vi "ModeMgr.Load Mode Config.vi"(6 "Options":string[](array[string])=["Display Result Data Details", "Not Reset SN between Tests", "Not Validate Operator", "Not Validate SN", "Disable Results", "Can Access Station Module", "Can Edit EQ List", "Can Clear Warnings", "Can Clear Errors", "Can View Config", "Can Edit Options", "Can Select Sequence", "Can Generate Reports", "Disable Start with SN Entry", "Can Auto Repeat Sequence"], 8 "Use DIalog":bool, 9 "Path":path, 10 "Modes":T1[](array[typedef]) {"Color" items=["Red", "Yellow", "Orange", "Green", "SkyBlue", "Blue", "Purple", "Pink", "Grey"]}, 11 "Default Mode":string="Production") -> (0 "error out":errorcluster, 1 "Names":string[](array[string]), 2 "Modes Out":T1[](array[typedef]) {"Color" items=["Red", "Yellow", "Orange", "Green", "SkyBlue", "Blue", "Purple", "Pink", "Grey"]}, 3 "Default Mode Out":string="Production")   [LabVIEW 2018]
uses:
  ModeMgr.Mode Settings_Config View.ctl
  ModeMgr.Mode Settings.ctl
  ModeMgr.ModeConfig.ctl
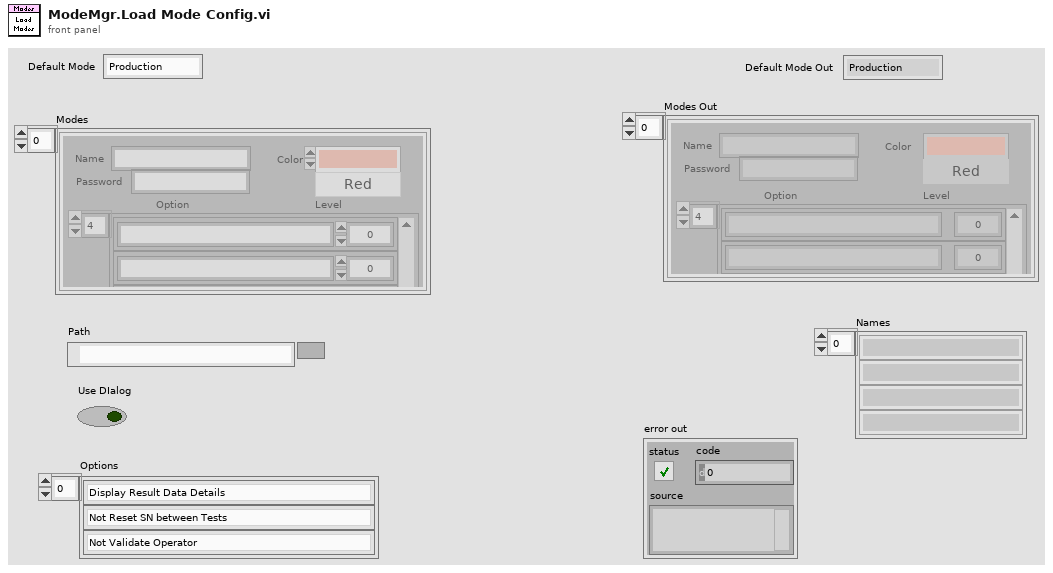
[diagram p1: front panel]
types:
  T1 = typedef "ModeMgr.Mode Settings_Config View.ctl" = cluster{"Name":string, "Color":u16, "Options":T2[], "Password":string}
  T2 = typedef "ModeMgr.Mode Settings.ctl" = cluster{"Option":string, "Level":i32}
  T3 = typedef "ModeMgr.ModeConfig.ctl" = cluster{"Name":string, "Color":string, "Settings":T2[], "Password":string}
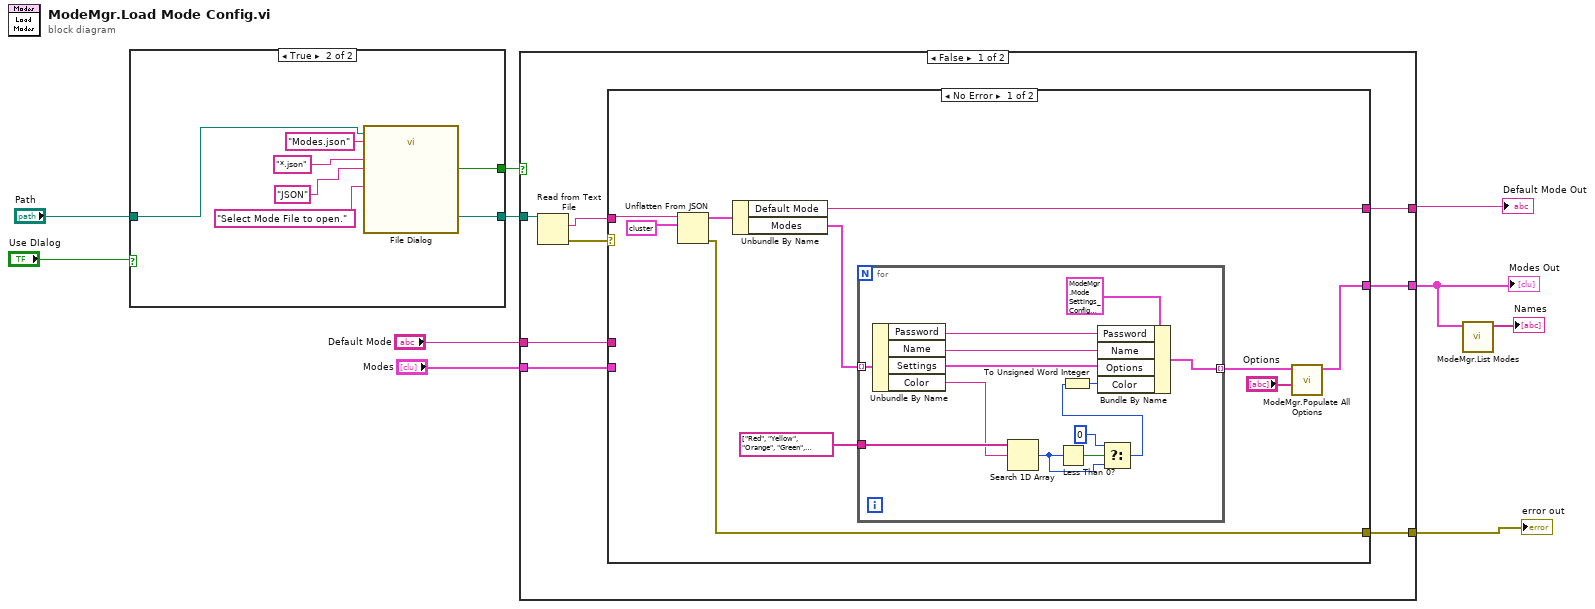
[diagram p0: block diagram]
diagram:
  n1 = case shown="True" "Use DIalog" {
    tunnel: [w11 w14] -> w10
    tunnel: "Path" -> [w11 w13]
    tunnel: [_ w12] -> w8
    frame False {
    }
    frame True {
      n2 = call "File Dialog"("start path"=w13, "prompt"="Select Mode File to open." ("prompt (Choose or enter file path)"), "default name"="Modes.json", "pattern (all files)"="*.json", "pattern label"="JSON" ("pattern (all files)")) -> ("selected path"=w14:path, "cancelled"=w12:bool)  [unwired: 7 in, 2 out]
    }
  }
  n3 = case shown="False" w8 {
    tunnel: w10 -> [w25 _]
    tunnel: [w24 w53] -> w6
    tunnel: [w23 w52] -> w3
    tunnel: "Default Mode" -> [w22 w53]
    tunnel: "Modes" -> [w21 w52]
    tunnel: [w19 _] -> w1
    frame False {
      n4 = Read from Text File(file (use dialog)=w25) -> (text=w26:string, error out=w20:errorcluster)  [unwired: 3 in, 2 out]
      n5 = case shown="No Error" w20 {
        tunnel: w26 -> [w36 _]
        tunnel: [w31 _] -> w19
        tunnel: [w29 w51] -> w24
        tunnel: [w27 w50] -> w23
        tunnel: w22 -> [_ w51]
        tunnel: w21 -> [_ w50]
        frame No Error {
          n6 = Unflatten From JSON(JSON string=w36, type and defaults=cluster{"Default Mode":string, "Modes":T3[]} {"Default Mode"="Production", "Modes"=[{"Name"="Production", "Color"="Green", "Settings"=[{"Option"="PreTest_Validate_SN", "Level"=1}, {"Option"="PostTest_ReportResult", "Level"=1}, {"Option"="OptTo_NotSaveResults", "Level"=0}, {"Option"="OptTo_NotStopOnFail", "Level"=0}, {"Option"="OptTo_SetConfig", "Level"=0}, {"Option"="OptTo_UpdateEquipmentList", "Level"=0}, {"Option"="OptTo_AccessManualStaControl", "Level"=0}], "Password"=""}, {"Name"="Technician", "Color"="Yellow", "Settings"=[{"Option"="PreTest_Validate_SN", "Level"=0}, {"Option"="PostTest_ReportResult", "Level"=0}, {"Option"="OptTo_NotSaveResults", "Level"=1}, {"Option"="OptTo_NotStopOnFail", "Level"=1}, {"Option"="OptTo_SetConfig", "Level"=0}, {"Option"="OptTo_UpdateEquipmentList", "Level"=0}, {"Option"="OptTo_AccessManualStaControl", "Level"=0}], "Password"=""}, {"Name"="Engineering", "Color"="SkyBlue", "Settings"=[{"Option"="PreTest_Validate_SN", "Level"=0}, {"Option"="PostTest_ReportResult", "Level"=0}, {"Option"="OptTo_NotSaveResults", "Level"=1}, {"Option"="OptTo_NotStopOnFail", "Level"=1}, {"Option"="OptTo_SetConfig", "Level"=1}, {"Option"="OptTo_UpdateEquipmentList", "Level"=1}, {"Option"="OptTo_AccessManualStaControl", "Level"=1}], "Password"=""}, {"Name"="Production", "Color"="Green", "Settings"=[], "Password"=""}, {"Name"="Technician", "Color"="Yellow", "Settings"=[], "Password"=""}, {"Name"="Engineering", "Color"="Blue", "Settings"=[], "Password"=""}]} ("Mode Config")) -> (value=w34:cluster{"Default Mode":string, "Modes":T3[]}, error out=w31:errorcluster)  [unwired: 5 in]
          n7 = Unbundle By Name(w34) -> ("Default Mode"=w29:string, "Modes"=w33:T3[])
          n8 = for {
            tunnel: w33 -> [w49] mode=indexing
            tunnel: string[] ["Red", "Yellow", "Orange", "Green", "SkyBlue", "Blue", "Purple", "Pink", "Grey"] ("Names") -> [w46]
            tunnel: [w39] -> w28 mode=indexing
            n9 = Unbundle By Name(w49) -> ("Password"=w37:string, "Name"=w48:string, "Settings"=w47:T2[], "Color"=w45:string)
            n10 = Search 1D Array(1D array=w46, element=w45) -> (index of element=w43:i32)  [unwired: 1 in]
            n11 = Less Than 0?(x=w43) -> (x < 0?=w44:bool)
            n12 = Select(t=0, s=w44, f=w43) -> (s? t:f=w41:i32)
            n13 = To Unsigned Word Integer(number=w41) -> (unsigned 16bit integer=w40:u16)
            n14 = Bundle By Name(cluster=T1 {"Name"="Production", "Color"=3, "Options"=[{"Option"="Can Access Station Module", "Level"=0}, {"Option"="Can Clear Errors", "Level"=0}, {"Option"="Can Clear Warnings", "Level"=0}, {"Option"="Can Edit EQ List", "Level"=0}, {"Option"="Can Edit Options", "Level"=0}, {"Option"="Can Generate Reports", "Level"=0}, {"Option"="Can Select Sequence", "Level"=0}, {"Option"="Can View Config", "Level"=0}, {"Option"="Disable Results", "Level"=0}, {"Option"="Disable Start with SN Entry", "Level"=0}, {"Option"="Display Result Data Details", "Level"=0}, {"Option"="Not Reset SN between Tests", "Level"=0}, {"Option"="Not Validate Operator", "Level"=0}, {"Option"="Not Validate SN", "Level"=0}], "Password"=""} ("Config"), "Password"=w37, "Name"=w48, "Options"=w47, "Color"=w40) -> (w39:T1)
          }
          n15 = call "ModeMgr.Populate All Options.vi"("Options"="Options", "Modes"=w28) -> ("Modes Out"=w27:T1[])  [unwired: 9 in]
        }
        frame Error {
          # "Do nothing.  No File"
        }
      }
    }
    frame True {
      # "Canceled"
    }
  }
  "Default Mode Out" <- w6
  "Modes Out" <- w3
  "error out" <- w1
  n16 = call "ModeMgr.List Modes.vi"("Modes"=w3) -> ("Names"=→"Names":string[])  [unwired: 10 in]
